vi "Update Z Cursors.vi"(8 "error in (no error)":errorcluster, 11 "Analysis Graph in":refnum<class "Analysis Graph.lvclass">) -> (0 "error out":errorcluster, 3 "Analysis Graph out":refnum<class "Analysis Graph.lvclass">)   [LabVIEW 2023, in "Analysis Graph.lvclass"]
uses:
  Analysis Graph.lvclass
  D:/git/Graph-Classes/Series Graph/Series Graph.lvclass
  Series Graph/Series Graph.lvclass/Series Graph.ctl
  Analysis Graph.lvclass/Analysis Graph.ctl
  Series Graph/Series Graph.lvclass
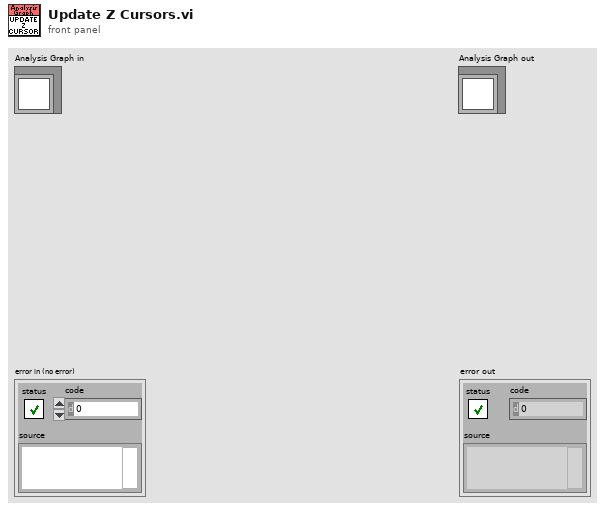
[diagram p1: front panel]
types:
  T1 = cluster{"ROI X":cluster{"Index":u32, "Length":u32}, "ROI Y":cluster{"Index":u32, "Length":u32}, "ROI Z":cluster{"Index":u32, "Length":u32}}
  T2 = typedef "LVCursorListTypeDef.ctl" = cluster{"Name":string, "Color":u32, "Style":u8, "Point Style":u8, "Name Visible":bool, "Allow Drag":bool, "Cursor Mode":u32, "Plot":i32, "Index":i32, "Position":cluster{"X":dbl, "Y":dbl}, "X Scale":u32, "Y Scale":u32, "Watch Plots":i32[], "Watch All Plots":bool, "Plot Area":i32, "Label Offset":cluster{"X":dbl, "Y":dbl}}[]
  T3 = cluster{"Name":string, "Color":u32, "Style":u8, "Point Style":u8, "Name Visible":bool, "Allow Drag":bool, "Cursor Mode":u32, "Plot":i32, "Index":i32, "Position":cluster{"X":dbl, "Y":dbl}, "X Scale":u32, "Y Scale":u32, "Watch Plots":i32[], "Watch All Plots":bool, "Plot Area":i32, "Label Offset":cluster{"X":dbl, "Y":dbl}}
  T4 = cluster{"Name":string, "Color":u32, "Style":u8, "Point Style":u8, "Name Visible":bool, "Allow Drag":bool, "Cursor Mode":u32, "Plot":i32, "Index":i32, "Position":cluster{"X":dbl, "Y":dbl}, "X Scale":u32, "Y Scale":u32, "Watch Plots":i32[], "Watch All Plots":bool, "Plot Area":i32, "Label Offset":cluster{"X":dbl, "Y":dbl}}[]
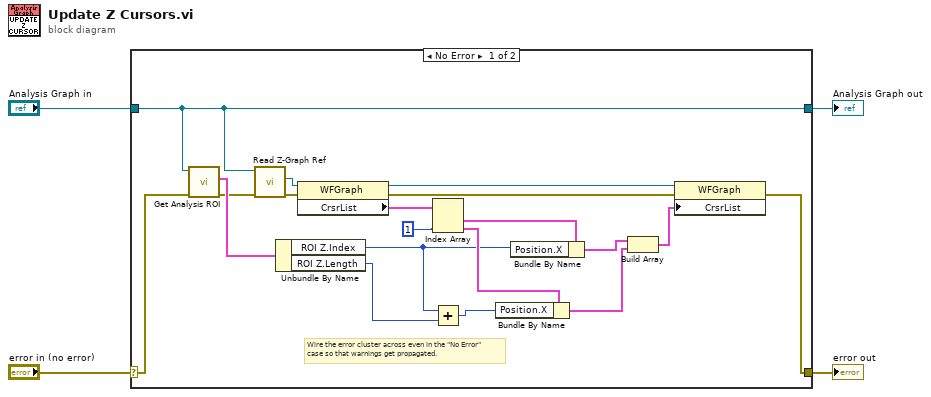
[diagram p0: block diagram]
diagram:
  n1 = case shown="No Error" "error in (no error)" {
    selector: "error in (no error)" -> [w23 w25]
    tunnel: [w7 w25] -> w3
    tunnel: [w21 w24] -> w1
    tunnel: "Analysis Graph in" -> [w21 w24]
    frame No Error {
      # "Wire the error cluster across even in the \"No Error\"\ncase so that warnings get propagated."
      n2 = call "Get Analysis ROI.vi"("error in (no error)"=w23, "Analysis Graph in"=w21) -> ("error out"=w20:errorcluster, "ROI XYZ"=w22:T1)  [unwired: 7 in, 1 out]
      n3 = call "Read Z-Graph Ref.vi"("error in (no error)"=w20, "Series Graph in"=w21) -> ("error out"=w18:errorcluster, "Z-Graph Ref"=w19:refnum<vi>)  [unwired: 7 in, 1 out]
      n4 = Unbundle By Name(w22) -> ("ROI Z.Index"=w5:u32, "ROI Z.Length"=w13:u32)
      n5 = property class="WFGraph"(reference=w19, error in=w18) -> (reference out=w12:refnum<vi>, error out=w11:errorcluster, "CrsrList"=w17:T2)
      n6 = Index Array(array=w17, index #2=1 ("index")) -> (element #1=w15:T3, element #2=w14:T3)  [unwired: 1 in]
      n7 = Add(x=w5, y=w13) -> (x+y=w6:u32)
      n8 = Bundle By Name(cluster=w14, "Position.X"=w6) -> (w9:T3)
      n9 = Bundle By Name(cluster=w15, "Position.X"=w5) -> (w10:T3)
      n10 = Build Array(w10, w9) -> (w8:T4)
      n11 = property class="WFGraph"(reference=w12, error in=w11, "CrsrList"=w8) -> (error out=w7:errorcluster)  [unwired: 1 out]
    }
    frame Error {
    }
  }
  "error out" <- w3
  "Analysis Graph out" <- w1
